vi "0-Draw No-Sail Zones.vi"(4 "Image Descriptor":T2={"Upper-Left Corner Coordinates"={"UTM Zone"=0.0, "Hemisphere"=enum."North", "East"=0.0, "North"=0.0}, "Meters/Pixel"=42.294203} {"Upper-Left Corner Coordinates"."North" format="%#_10f"; "Upper-Left Corner Coordinates"."East" format="%#_8f"}, 6 "No Sail Circles":T1[](array[typedef]), 7 "Image In":T4) -> (1 "Coordinate Outside Image":bool, 3 "Image Out":T4)   [LabVIEW 2011]
doc: "Overlays no-sail zones onto the map image.\nTODO: make graphical repr nicer"
uses:
  <vilib>/vision/Image Controls.llb/IMAQ Image.ctl
  0-Image Descriptor.ctl
  2-Think/2 Typedefs/UTM Location.ctl
  2-Think/2 Typedefs/UTM Circle.ctl
panel:
  in  "No Sail Zone Color":u32(colorbox)=16754450
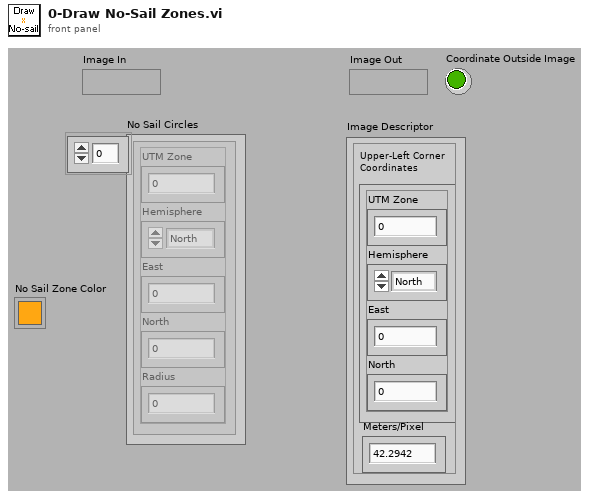
[diagram p1: front panel]
types:
  T1 = typedef "UTM Circle.ctl" = cluster{"UTM Zone":dbl, "Hemisphere":enum16{"North", "South"}, "East":dbl, "North":dbl, "Radius":dbl}
  T2 = typedef "0-Image Descriptor.ctl" = cluster{"Upper-Left Corner Coordinates":T3, "Meters/Pixel":dbl}
  T3 = typedef "UTM Location.ctl" = cluster{"UTM Zone":dbl, "Hemisphere":enum16{"North", "South"}, "East":dbl, "North":dbl}
  T4 = typedef "IMAQ Image.ctl" = refnum<image>
  T5 = cluster{"Desired Font (Application)":enum16{"User-specified Font", "Application Font", "System Font", "Dialog Font"}, "[User-specified Font]":cluster{"Font Name":string, "Size":i16, "Strikeout?":bool, "Italic?":bool, "Underline?":bool, "Outline?":bool, "Shadow?":bool, "Bold?":bool, "Rotation Angle":dbl}, "Horizontal Alignment":i16, "Vertical Alignment":i16}
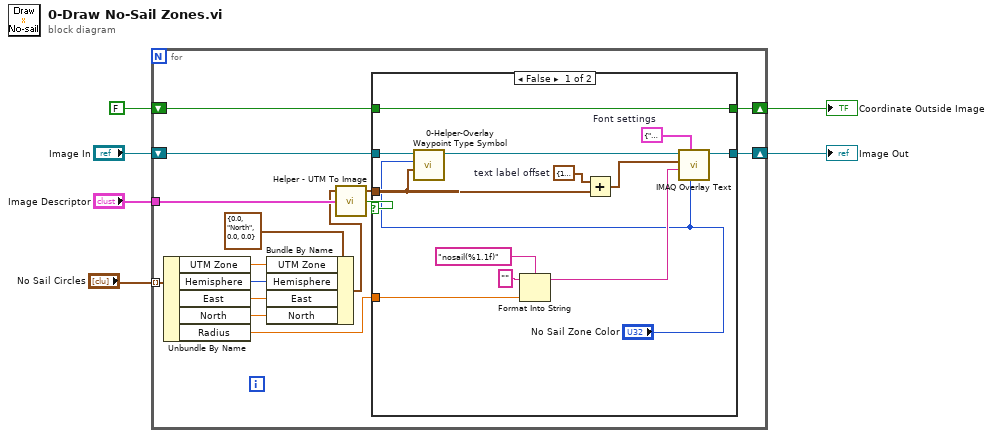
[diagram p0: block diagram]
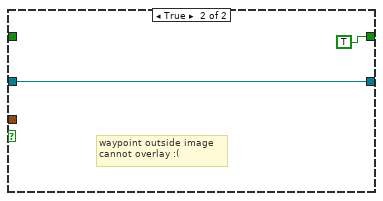
[diagram p2: hidden frame]
diagram:
  n1 = for {
    tunnel: "No Sail Circles" -> [w14] mode=indexing
    shift-right: [w20] -> w5
    shift-left: "Image In" -> [w21]
    tunnel: "Image Descriptor" -> [w19]
    shift-right: [w16] -> w3
    shift-left: FALSE -> [w15]
    n2 = Unbundle By Name(w14) -> ("UTM Zone"=w8:dbl, "Hemisphere"=w9:enum16{"North", "South"}, "East"=w10:dbl, "North"=w11:dbl, "Radius"=w13:dbl)
    n3 = Bundle By Name(cluster=T3 {"UTM Zone"=0.0, "Hemisphere"=enum."North", "East"=0.0, "North"=0.0} ("UTM Location"), "UTM Zone"=w8, "Hemisphere"=w9, "East"=w10, "North"=w11) -> (w7:T3)
    n4 = call "Helper - UTM To Image.vi"("Image Descriptor"=w19, "UTM Location"=w7) -> ("Coordinate Outside Image"=w17:bool, "Pixel Coordinates"=w18:cluster{"X":i32, "Y":i32})  [unwired: 1 in, 1 out]
    n5 = case shown="False" w17 {
      tunnel: w21 -> [w26 w36]
      tunnel: [w31 w36] -> w20
      tunnel: w18 -> [w25 _]
      tunnel: [w28 TRUE] -> w16
      tunnel: w15 -> [w28 _]
      tunnel: w13 -> [w22 _]
      frame False {
        w34 = T5 {"Desired Font (Application)"=enum."User-specified Font", "[User-specified Font]"={"Font Name"="Arial Unicode MS", "Size"=40, "Strikeout?"=FALSE, "Italic?"=FALSE, "Underline?"=FALSE, "Outline?"=FALSE, "Shadow?"=FALSE, "Bold?"=TRUE, "Rotation Angle"=0.0}, "Horizontal Alignment"=0, "Vertical Alignment"=0}  # Font settings
        w33 = cluster{"X":i32, "Y":i32} {"X"=10, "Y"=21}  # text label offset
        n6 = call "0-Helper-Overlay Waypoint Type Symbol.vi"("Overlay Location"=w25, "Icon Color"="No Sail Zone Color", "Image in"=w26) -> ("Image out"=w27:T4)  [unwired: 7 in, 1 out]
        n7 = Format Into String(format string="nosail(%1.1f)", initial string="", w22) -> (resulting string=w29:string)  [unwired: 1 in, 1 out]
        n8 = Add(x=w33, y=w25) -> (x+y=w32:cluster{"X":i32, "Y":i32})
        n9 = call "IMAQ Overlay Text"("Text Color (black)"="No Sail Zone Color", "Font, Size & Style"=w34, "String"=w29, "Origin"=w32, "Image"=w27) -> ("Image Out"=w31:T4)  [unwired: 3 in, 3 out]
      }
      frame True {
        # "waypoint outside image\ncannot overlay :("
      }
    }
  }
  "Image Out" <- w5
  "Coordinate Outside Image" <- w3
